vi "train_get.vi"(7 "LabVIEW Web Service Request":refnum<class "Web Request.lvclass">) -> ()   [LabVIEW 2014]
uses:
  <vilib>/wsapi/Web Request.lvclass
  DataManager/StateStore/Controls/DataFunction.ctl
panel:
  out "timing":u32
  out "error out 2":errorcluster
  out "error out":errorcluster
  # "Use the Web Service Request input terminal to call the VIs on the Web Services palette. Do not remove it from the connector pane unless you don't need access to the palette."
  # "Each additional control wired to the connector pane will be available as an input in the URL. To include an indicator in terminal-mode output (the default setting), it must also be wired to the connector pane."
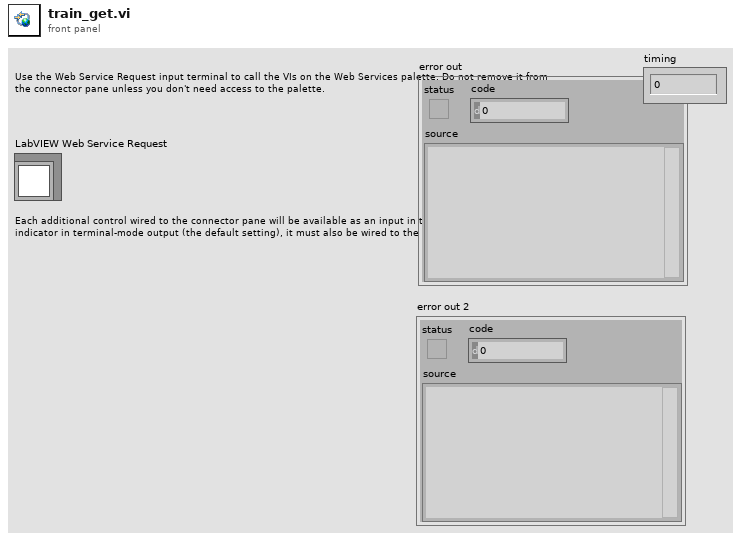
[diagram p1: front panel]
types:
  T1 = cluster{"uuid":string, "throttle":dbl, "brake":dbl, "horn":dbl, "wait":dbl, "name":string, "mode":string, "dest":string}
  T2 = typedef "DataFunction.ctl" = enum16{"Initialise", "Release", "Get Data", "Set Data", "Preview Data"}
  T3 = typedef "CData Core Control.ctl" = cluster{"train_data_array":cluster{"uuid":string, "int":i32, "posit_array":cluster{"x":dbl, "y":dbl, "z":dbl}[]}[], "train_control_array":cluster{"uuid":string, "throttle":dbl, "brake":dbl, "horn":dbl, "wait":dbl, "name":string, "mode":string, "dest":string}[], "switch_data_array":cluster{"switch_posit":cluster{"x":dbl, "y":dbl, "z":dbl}, "manual":bool}[], "switch_control_array":cluster{"switch_posit":cluster{"x":dbl, "y":dbl, "z":dbl}, "switch":bool, "invert":bool, "wait":dbl}[]}
  T4 = cluster{"uuid":string, "throttle":dbl, "brake":dbl, "horn":dbl, "wait":dbl, "name":string, "mode":string, "dest":string}[]
  T5 = cluster{"0":string, "1":dbl, "2":dbl, "3":dbl, "4":dbl, "5":string, "6":string, "7":string}
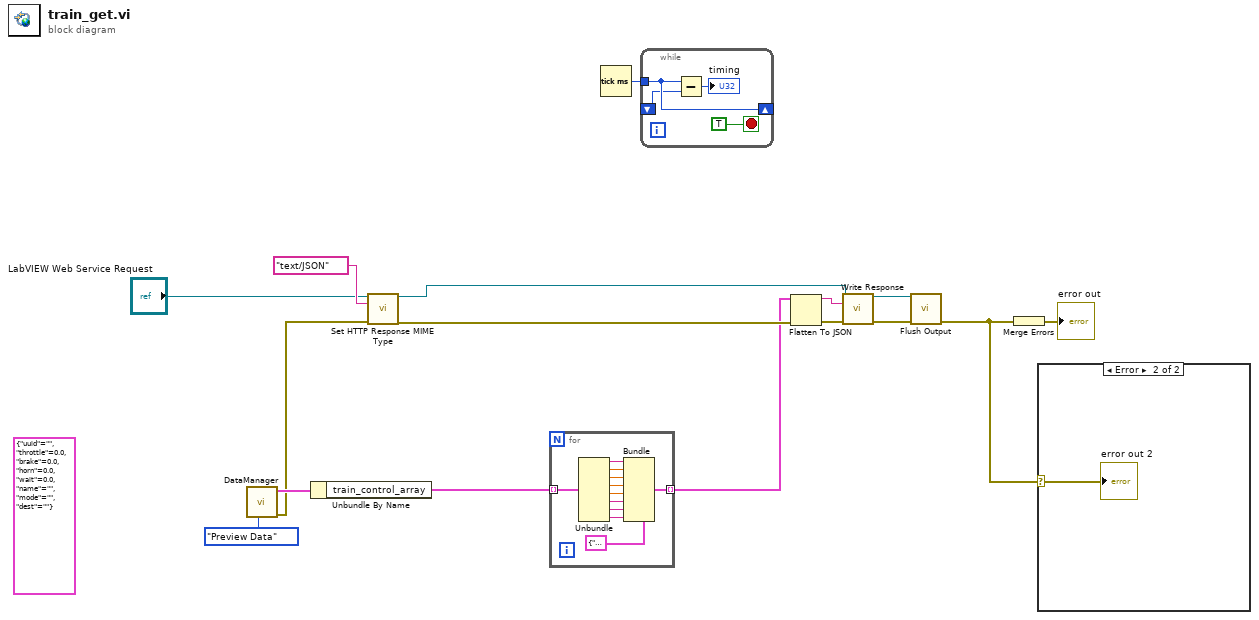
[diagram p0: block diagram]
diagram:
  (unwired) T1 {"uuid"="", "throttle"=0.0, "brake"=0.0, "horn"=0.0, "wait"=0.0, "name"="", "mode"="", "dest"=""} ("train_control")
  n1 = call "DataManager.vi"("DataFunction"=DataFunction."Preview Data") -> ("error out"=w5:errorcluster, "CData Out"=w8:T3)  [unwired: 9 in]
  n2 = Unbundle By Name(w8) -> ("train_control_array"=w2:T4)
  n3 = call <vilib>:"Set HTTP Response MIME Type.vi"("LabVIEW Web Service Request"="LabVIEW Web Service Request", "MIME type (text/html)"="text/JSON", "error in (no error)"=w5) -> ("LabVIEW Web Service Request out"=w10:refnum<class "Web Request.lvclass">, "error out"=w6:errorcluster)  [unwired: 11 in]
  n4 = for {
    tunnel: w2 -> [w27] mode=indexing
    tunnel: [w18] -> w1 mode=indexing
    n5 = Unbundle(w27) -> ("uuid"=w19:string, "throttle"=w20:dbl, "brake"=w21:dbl, "horn"=w22:dbl, "wait"=w23:dbl, "name"=w24:string, "mode"=w25:string, "dest"=w26:string)
    n6 = Bundle(cluster=T5 {"0"="", "1"=0.0, "2"=0.0, "3"=0.0, "4"=0.0, "5"="", "6"="", "7"=""} ("train_control"), "0"=w19, "1"=w20, "2"=w21, "3"=w22, "4"=w23, "5"=w24, "6"=w25, "7"=w26) -> (w18:T5)
  }
  n7 = Tick Count (ms)() -> (millisecond timer value=w3:u32)
  n8 = while {
    tunnel: w3 -> [w31]
    shift-right: [w31] -> _
    shift-left: _ -> [w30]
    stop <- TRUE stop-if-true
    n9 = Subtract(x=w31, y=w30) -> (x-y=→"timing":u32)
  }
  n10 = Flatten To JSON(anything=w1, error in (no error)=w6) -> (JSON string=w16:string, 11:w7:errorcluster)  [unwired: 1 in]
  n11 = call <vilib>:"Write Response.vi"("LabVIEW Web Service Request"=w10, "response string"=w16, "error in (no error)"=w7) -> ("LabVIEW Web Service Request out"=w14:refnum<class "Web Request.lvclass">, "error out"=w13:errorcluster)  [unwired: 11 in]
  n12 = call <vilib>:"Flush Output.vi"("LabVIEW Web Service Request"=w14, "error in (no error)"=w13) -> ("error out"=w4:errorcluster)  [unwired: 12 in, 1 out]
  n13 = Merge Errors(w4) -> (→"error out":errorcluster)
  n14 = case shown="Error" w4 {
    selector: w4 -> [_ w32]
    frame No Error {
    }
    frame Error {
      "error out 2" <- w32
    }
  }
